vi "rad_NI-Auth Login Dialog.vi"(8 "error in (no error)":errorcluster, 11 "Target Address":string="10.0.19.46") -> (0 "error out":errorcluster, 1 "Cancelled":bool, 2 "Password Out":string, 3 "session out":refnum<k21>)   [LabVIEW 2016]
uses:
  Util/FP Control/FP Control Functions.ctl
  <vilib>/nisyscfg/Close (System).vi
  <vilib>/nisyscfg/nisyscfg.lvlib
panel:
  out "Target":string
  in  "Cancel":bool
  in  "OK":bool
  in  "Password:":string
  # "Permission required for:"
  # "User Name: admin"
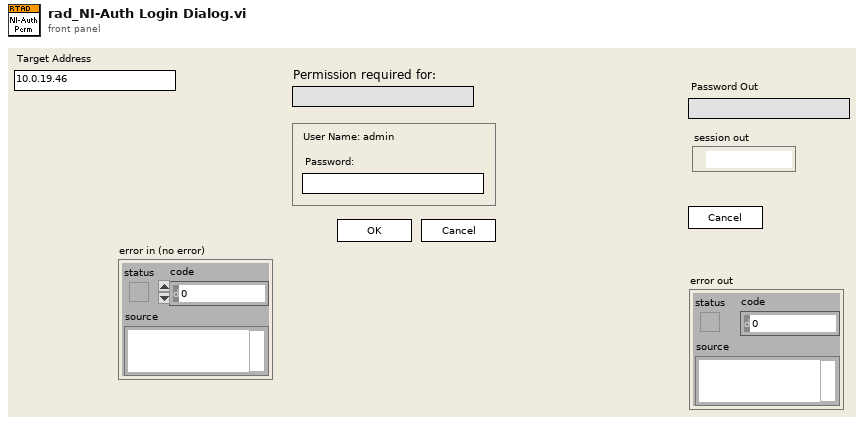
[diagram p1: front panel]
types:
  T1 = typedef "FP Control Functions.ctl" = enum16{"Open", "Close", "Bring To Front", "Center"}
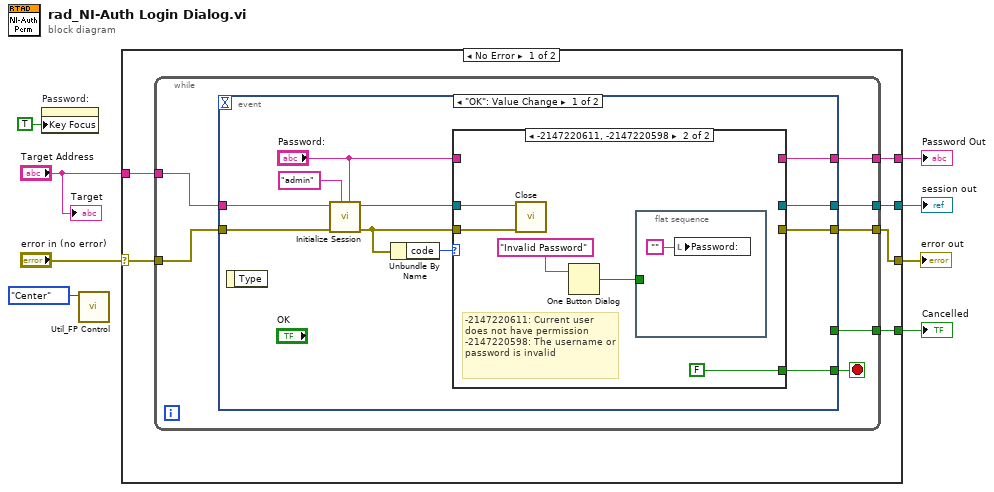
[diagram p0: block diagram]
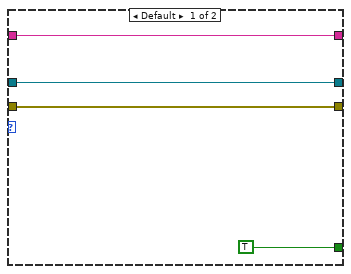
[diagram p2: hidden frame]
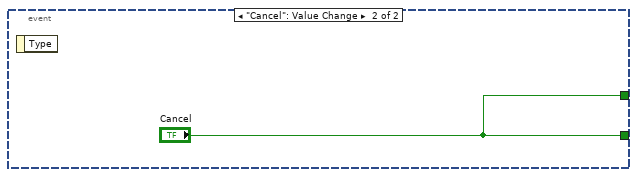
[diagram p3: hidden frame]
diagram:
  n1 = property on="Password:" class="Str"("Key Focus"=TRUE) -> ()  [unwired: 2 in, 2 out]
  n2 = call "Util_FP Control.vi"("Function"=FP_Control_Functions."Center") -> ()  [unwired: 10 in, 1 out]
  n3 = case shown="No Error" "error in (no error)" {
    selector: "error in (no error)" -> [w9 w44]
    tunnel: "Target Address" -> [w14 _]
    tunnel: [w13 w44] -> w8
    tunnel: [w12 _] -> w7
    tunnel: [w11 _] -> w6
    tunnel: [w10 _] -> w5
    frame No Error {
      n4 = while {
        tunnel: w14 -> [w21]
        tunnel: [w19] -> w13
        tunnel: [w18] -> w12
        tunnel: [w17] -> w11
        tunnel: [w16] -> w10
        tunnel: w9 -> [w15]
        stop <- w20 stop-if-true
        n5 = event shown="[0] \"OK\": Value Change" {
          selector: _ -> [_ _]
          dyn-events: _ -> [_ _]
          timeout: _ -> [_ _]
          tunnel: w21 -> [w31 _]
          tunnel: [w29 "Cancel"] -> w20
          tunnel: [w27 _] -> w19
          tunnel: [w25 _] -> w18
          tunnel: [w23 _] -> w17
          tunnel: [_ "Cancel"] -> w16
          tunnel: w15 -> [w22 _]
          event "OK": Value Change {
            n6 = event-data() -> ()  [unwired: 1 in, 1 out]
            n7 = call <vilib>:"Initialize Session.vi"("Password"="Password:", "User Name"="admin" ("user name"), "error in (no error)"=w22, "Target (localhost)"=w31) -> ("error out"=w28:errorcluster, "Session out"=w24:refnum<k21>)  [unwired: 6 in]
            n8 = Unbundle By Name(w28) -> ("code"=w30:i32)
            n9 = case shown="-2147220611, -2147220598" w30 {
              tunnel: [TRUE FALSE] -> w29
              tunnel: w28 -> [w36 w38]
              tunnel: [w36 _] -> w27
              tunnel: "Password:" -> [w35 _]
              tunnel: [w35 _] -> w25
              tunnel: w24 -> [w33 w39]
              tunnel: [w33 _] -> w23
              frame Default {
              }
              frame -2147220611, -2147220598 {
                # "-2147220611: Current user does not have permission\n-2147220598: The username or password is invalid"
                n10 = call-poly <vilib>:"Close.vi"("error in (no error)"=w38, "Session in"=w39) -> ()  [unwired: 9 in, 1 out]
                n11 = One Button Dialog(message="Invalid Password") -> (true=w37:bool)  [unwired: 1 in]
                n12 = flat-sequence {
                  tunnel: w37 -> [_]
                  frame #0 {
                    n13 = local write "Password:"("" ("Password:")) -> ()
                  }
                }
              }
            }
          }
          event "Cancel": Value Change {
            n14 = event-data() -> ()  [unwired: 1 in, 1 out]
          }
        }
      }
    }
    frame Error {
    }
  }
  "Password Out" <- w7
  "Cancelled" <- w5
  "error out" <- w8
  "session out" <- w6
  "Target" <- "Target Address"
